vi "DisplayGrid.vi"(9 "Grid":T1, 11 "input picture":picture) -> (3 "new picture":picture)   [LabVIEW 2020]
uses:
  Global Variables/Global Correct Answer.vi
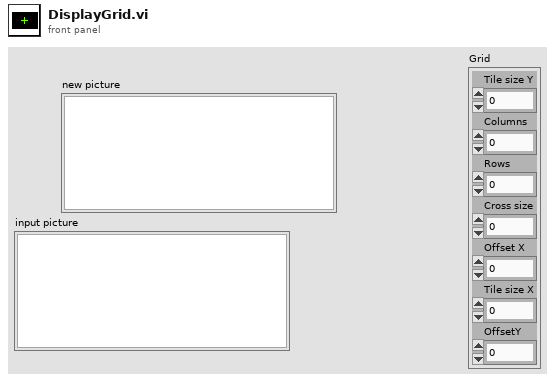
[diagram p1: front panel]
types:
  T1 = cluster{"Tile size Y":dbl, "Columns":dbl, "Rows":dbl, "Cross size":dbl, "Offset X":dbl, "Tile size X":dbl, "OffsetY":dbl}
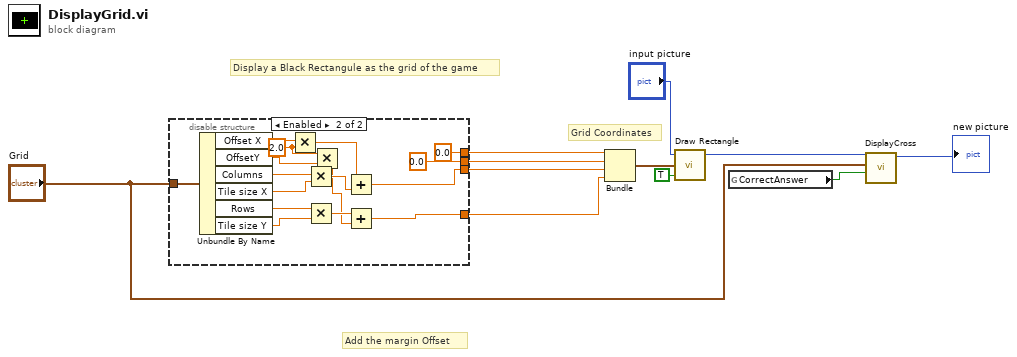
[diagram p0: block diagram]
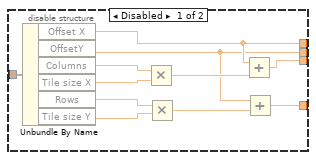
[diagram p2: hidden frame]
diagram:
  # "Grid Coordinates"
  # "Add the margin Offset"
  # "Display a Black Rectangule as the grid of the game"
  n1 = disable-structure shown="Enabled" {
    disable-tunnel: "Grid" -> [w22 w38]
    disable-tunnel: [w16 0.0 ("Offset X")] -> w4
    disable-tunnel: [w15 w35] -> w3
    disable-tunnel: [w13 0.0 ("OffsetY")] -> w2
    disable-tunnel: [w12 w34] -> w1
    frame Disabled {
      n2 = Unbundle By Name(w22) -> ("Offset X"=w16:dbl, "OffsetY"=w13:dbl, "Columns"=w18:dbl, "Tile size X"=w19:dbl, "Rows"=w20:dbl, "Tile size Y"=w21:dbl)
      n3 = Multiply(x=w18, y=w19) -> (x*y=w17:dbl)
      n4 = Multiply(x=w20, y=w21) -> (x*y=w14:dbl)
      n5 = Add(x=w16, y=w17) -> (x+y=w15:dbl)
      n6 = Add(x=w13, y=w14) -> (x+y=w12:dbl)
    }
    frame Enabled {
      w25 = 2.0 ("y")
      n7 = Unbundle By Name(w38) -> ("Offset X"=w27:dbl, "OffsetY"=w26:dbl, "Columns"=w29:dbl, "Tile size X"=w30:dbl, "Rows"=w31:dbl, "Tile size Y"=w32:dbl)
      n8 = Multiply(x=w27, y=w25) -> (x*y=w24:dbl)
      n9 = Multiply(x=w29, y=w30) -> (x*y=w28:dbl)
      n10 = Multiply(x=w31, y=w32) -> (x*y=w33:dbl)
      n11 = Multiply(x=w25, y=w26) -> (x*y=w23:dbl)
      n12 = Add(x=w24, y=w28) -> (x+y=w35:dbl)
      n13 = Add(x=w33, y=w23) -> (x+y=w34:dbl)
    }
  }
  n14 = Bundle("Offset X"=w4, "OffsetY"=w2, w3, w1) -> (w10:cluster{"Offset X":dbl, "OffsetY":dbl, dbl, dbl})  [unwired: 1 in]
  n15 = call <vilib>:"Draw Rectangle.vi"("picture"="input picture", "rect"=w10, "fill?(F)"=TRUE) -> ("new picture"=w8:picture)  [unwired: 6 in]
  n16 = global read "Global Correct Answer.vi" "CorrectAnswer"() -> (w6:bool)
  n17 = call "DisplayCross.vi"("CorrectAnswer"=w6, "Grid"="Grid", "new picture in"=w8) -> ("new picture out"=→"new picture":picture)  [unwired: 8 in]
